vi "ep_Torque Load Efficiency (1 Chan).vi"(0 "phase voltage waveforms":waveform(dbl)[](array[waveform]), 1 "current waveforms":waveform(dbl)[](array[waveform]), 2 "speed [RPM]":dbl, 3 "nominal frequency":enum16{"50 Hz", "60 Hz"}(ring), 4 "motor information":T2, 5 "error in (no error)":errorcluster, 6 "fundamental frequency [Hz]":dbl=50.0, 7 "initial conditions":T1, 8 "reset? (F)":bool, 9 "total input active power [W]":dbl, 11 "stator resistance [ohms]":dbl) -> (12 "torque waveform [Nm]":waveform(dbl), 13 "final conditions":T1, 14 "torque [Nm]":dbl, 15 "load [kW]":dbl, 16 "efficiency [%]":dbl, 19 "error out":errorcluster)   [LabVIEW 2014, in "NI_EP_Motor Monitoring.lvlib"]
uses:
  <vilib>/addons/Electrical Power/Motor Monitoring/NI_EP_Motor Monitoring.lvlib
  <vilib>/addons/Electrical Power/Motor Monitoring/subVIs/ep_Initial Conditions for Air Gap.ctl
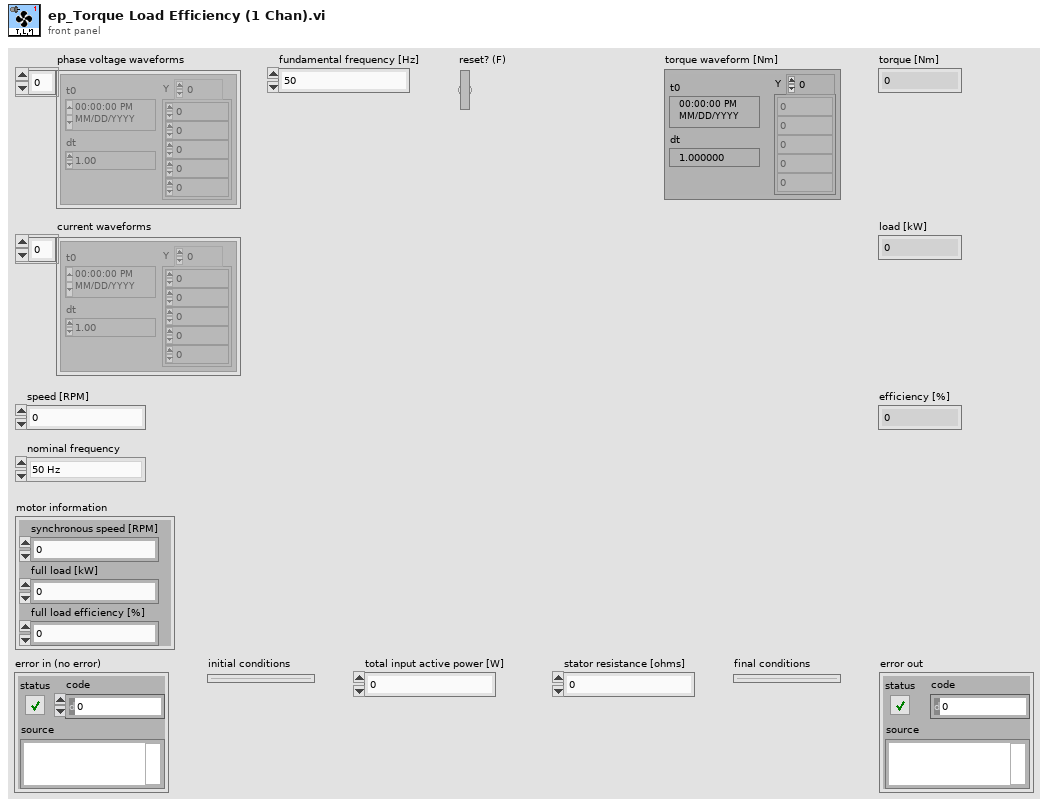
[diagram p1: front panel]
types:
  T1 = typedef "NI_EP_Motor Monitoring.lvlib/ep_Initial Conditions for Air Gap.ctl" = cluster{"integration state in A":cluster{"initial value":dbl, "initial integration":dbl}, "integration state in B":cluster{"initial value":dbl, "initial integration":dbl}, "integrated state A":dbl[], "integrated state B":dbl[], "previous length":i32, "loss and polepair":cluster{"Pstray [W]":dbl, "Pfric [W]":dbl, "Polepair #":i32, "synchronous speed [RPM]":dbl}, "expected timestamp":timestamp}
  T2 = cluster{"synchronous speed [RPM]":dbl, "full load [kW]":dbl, "full load efficiency [%]":dbl}
  T3 = cluster{"Pstray [W]":dbl, "Pfric [W]":dbl, "Polepair #":i32, "synchronous speed [RPM]":dbl}
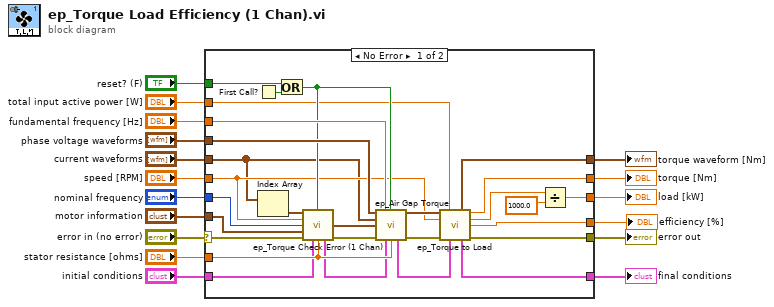
[diagram p0: block diagram]
diagram:
  n1 = case shown="No Error" "error in (no error)" {
    selector: "error in (no error)" -> [w45 w46]
    tunnel: [w35 w46] -> w16
    tunnel: "total input active power [W]" -> [w27 _]
    tunnel: "stator resistance [ohms]" -> [w38 _]
    tunnel: "motor information" -> [w26 _]
    tunnel: "nominal frequency" -> [w25 _]
    tunnel: "speed [RPM]" -> [w24 _]
    tunnel: "reset? (F)" -> [w43 _]
    tunnel: "current waveforms" -> [w22 _]
    tunnel: "phase voltage waveforms" -> [w41 _]
    tunnel: "fundamental frequency [Hz]" -> [w40 _]
    tunnel: [w34 _] -> w6
    tunnel: [w19 _] -> w5
    tunnel: [w32 _] -> w4
    tunnel: [w30 _] -> w3
    tunnel: "initial conditions" -> [w21 _]
    tunnel: [w28 _] -> w2
    frame No Error {
      n2 = First Call?() -> (First Call?: T/F=w44:bool)
      n3 = Index Array(array=w22) -> (element=w23:waveform(dbl))  [unwired: 1 in]
      n4 = Or(x=w43, y=w44) -> (x .or. y?=w39:bool)
      n5 = call <vilib>:"ep_Torque Check Error (1 Chan).vi"("signal"=w23, "reset? (F)"=w39, "speed [RPM]"=w24, "nominal frequency"=w25, "motor information"=w26, "error in (no error)"=w45, "initial conditions"=w21, "stator resistance [ohms]"=w38) -> ("information"=w37:T3, "final conditions"=w20:T1, "error out"=w42:errorcluster)  [unwired: 5 in]
      n6 = call <vilib>:"ep_Air Gap Torque.vi"("phase voltage waveforms"=w41, "fundamental frequency [Hz]"=w40, "reset? (F)"=w39, "current waveforms"=w22, "information"=w37, "error in (no error)"=w42, "initial conditions"=w20, "stator resistance [ohms]"=w38) -> ("air-gap torque waveform [Nm]"=w31:waveform(dbl), "final conditions"=w29:T1, "error out"=w36:errorcluster)  [unwired: 5 in]
      n7 = call <vilib>:"ep_Torque to Load.vi"("air-gap torque waveform [Nm]"=w31, "total input active power [W]"=w27, "speed [RPM]"=w24, "error in (no error)"=w36, "initial conditions"=w29) -> ("torque waveform [Nm]"=w30:waveform(dbl), "torque [Nm]"=w32:dbl, "load [W]"=w33:dbl, "efficiency [%]"=w34:dbl, "final conditions"=w28:T1, "error out"=w35:errorcluster)  [unwired: 5 in]
      n8 = Divide(x=w33, y=1000.0) -> (x/y=w19:dbl)
    }
    frame Error {
    }
  }
  "error out" <- w16
  "torque [Nm]" <- w4
  "load [kW]" <- w5
  "efficiency [%]" <- w6
  "torque waveform [Nm]" <- w3
  "final conditions" <- w2
